vi "PartitionBuildArray.vi"(10 "rt fifo":refnum<k33>) -> (2 "NN Set":sgl[][](array[numeric]), 3 "NN Set Check":sgl[][](array[numeric]))   [LabVIEW 2020]
uses:
  Global Variables/Training_Status.vi
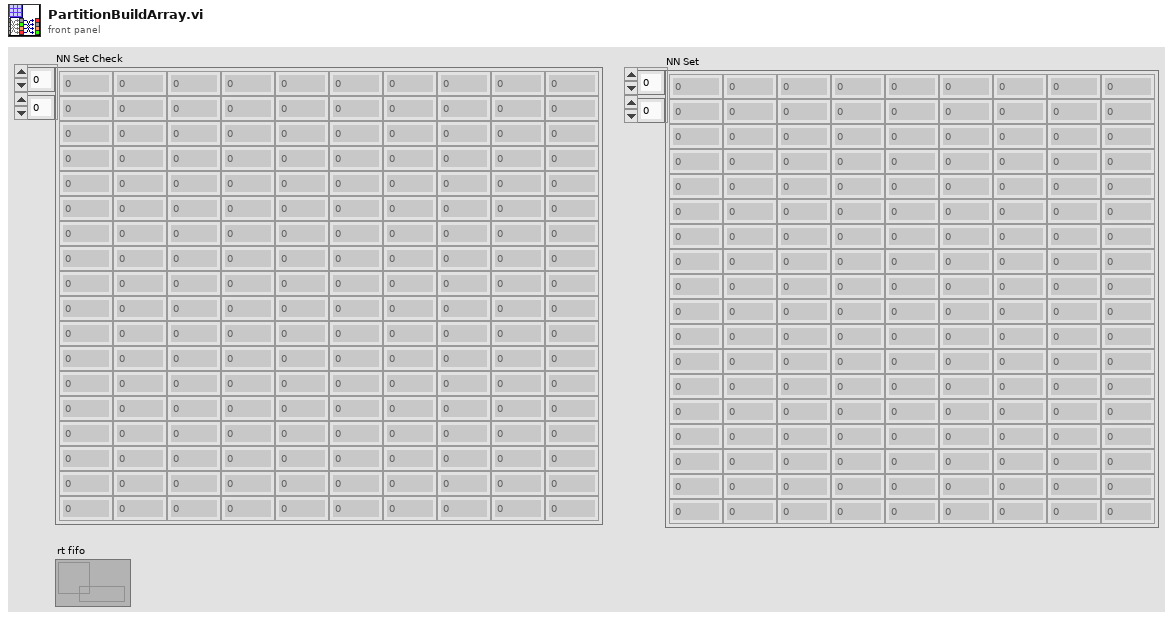
[diagram p1: front panel]
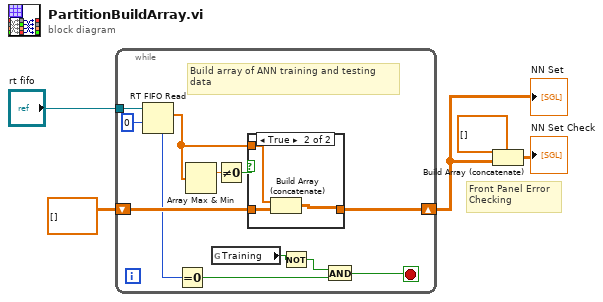
[diagram p0: block diagram]
diagram:
  # "Front Panel Error \nChecking"
  n1 = while {
    tunnel: "rt fifo" -> [w16]
    shift-right: [w14] -> w5
    shift-left: sgl[][] [] -> [w15]
    stop <- w9 stop-if-true
    # "Build array of ANN training and testing \ndata"
    n2 = RT FIFO Read(0:w16, 2:0 ("timeout in ms (0)")) -> (7:w10:u32, 9:w13:sgl[])  [unwired: 2 in, 3 out]
    n3 = Equal To 0?(x=w10) -> (x = 0?=w8:bool)
    n4 = Array Max & Min(array=w13) -> (max value=w11:sgl)  [unwired: 3 out]
    n5 = global read "Training_Status.vi" "Training"() -> (w6:bool)
    n6 = Not Equal To 0?(x=w11) -> (x != 0?=w12:bool)
    n7 = case shown="True" w12 {
      tunnel: w15 -> [w18 w21]
      tunnel: [w18 w20] -> w14
      tunnel: w13 -> [_ w19]
      frame False {
      }
      frame True {
        n8 = Build Array (concatenate)(w19, w21) -> (w20:sgl[][])
      }
    }
    n9 = Not(x=w6) -> (.not. x?=w7:bool)
    n10 = And(x=w7, y=w8) -> (x .and. y?=w9:bool)
  }
  "NN Set" <- w5
  n11 = Build Array (concatenate)(sgl[][] [] ("array"), w5) -> (→"NN Set Check":sgl[][])
